vi "Calculated Accuracy Parameter.vi"(0 "VISA resource name":refnum<visa-resource-name>, 7 "Temperature (5 C)":dbl=5.0 min=5.0 max=45.0 format="%.2f", 9 "Meas. Type (0:Z,Y)":enum16{"Z,Y", "L C X B", "R G"}(ring), 11 "error in (no error)":errorcluster) -> (3 "Frequency Used":dbl format="%.2f", 4 "VISA resource name out":refnum<visa-resource-name>, 8 "Ae Accuracy":dbl format="%.2f", 15 "error out":errorcluster)   [LabVIEW 2015, in "Agilent 428X Series.lvlib"]
doc: "This VI is to find the different Ae value for different measured.\n\nFor Z, Y, L, C, R, X, G and B accuracy:\nAe=[A+(Ka+Kaa+Kb*Kbb+Kc)*100+Kd]*Ke [%]\n\nDisclaimer: All accuracy calculation VI's are not part of the original \n driver. They are provided for supplementry purpose only.\n If user desires very high accuracy data, please do or \n check the calculation seperately."
uses:
  Agilent 428X Series.lvlib
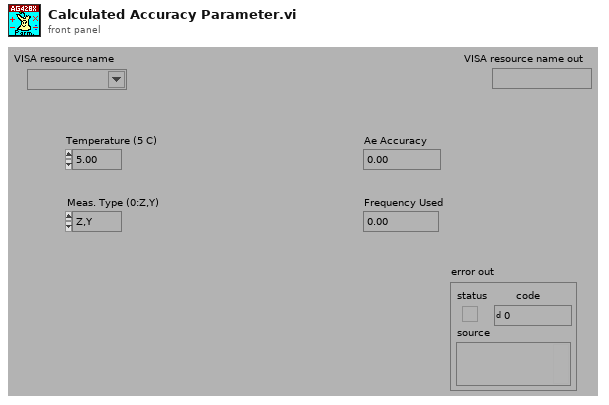
[diagram p1: front panel]
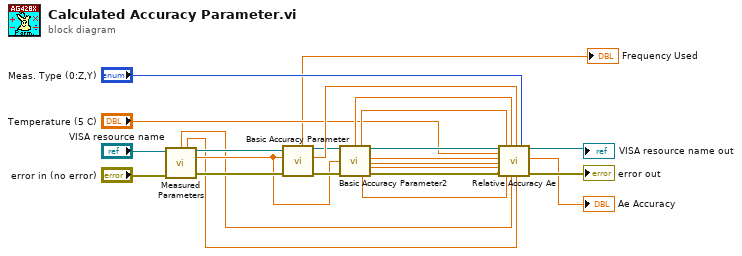
[diagram p0: block diagram]
diagram:
  n1 = call "Measured Parameters.vi"("VISA resource name"="VISA resource name", "error in (no error)"="error in (no error)") -> ("Dx"=w3:dbl, "Qx"=w2:dbl, "VISA resource name out"=w8:refnum<visa-resource-name>, "Z"=w6:dbl, "error out"=w7:errorcluster)  [unwired: 7 in, 2 out]
  n2 = call "Basic Accuracy Parameter.vi"("error in (no error)"=w7, "Impedance Z (10m)"=w6, "VISA resource name"=w8) -> ("error out"=w13:errorcluster, "Parameter A"=w19:dbl, "VISA resource name out"=w18:refnum<visa-resource-name>, "Frequency Used"=→"Frequency Used":dbl)  [unwired: 5 in]
  n3 = call "Basic Accuracy Parameter2.vi"("VISA resource name"=w18, "Impedance Z (10m)"=w6, "error in (no error)"=w13) -> ("Kbb"=w20:dbl, "Kaa"=w21:dbl, "VISA resource name out"=w17:refnum<visa-resource-name>, "Ka"=w24:dbl, "Kb"=w23:dbl, "Kc"=w22:dbl, "Kd"=w9:dbl, "error out"=w14:errorcluster)  [unwired: 5 in]
  n4 = call "Relative Accuracy Ae.vi"("VISA resource name"=w17, "Temperature (5 C)"="Temperature (5 C)", "Ka"=w24, "Kb"=w23, "Kc"=w22, "error in (no error)"=w14, "Kaa"=w21, "Kd"=w9, "Kbb"=w20, "Dx"=w3, "A"=w19, "Qx"=w2, "Meas. Type (0:Z,Y)"="Meas. Type (0:Z,Y)") -> ("VISA resource name out"=→"VISA resource name out":refnum<visa-resource-name>, "Ae Accuracy"=→"Ae Accuracy":dbl, "error out"=→"error out":errorcluster)  [unwired: 4 in]
